vi "niRFUtil MASMT Mean (DBL).vi"(8 "error in (no error)":errorcluster, 11 "X":dbl[](array[numeric])) -> (0 "error out":errorcluster, 3 "mean":dbl)   [LabVIEW 2015, in "niRFUtil.lvlib"]
doc: "Computes the mean value of the input sequence <B>X</B>."
uses:
  niRFUtil.lvlib
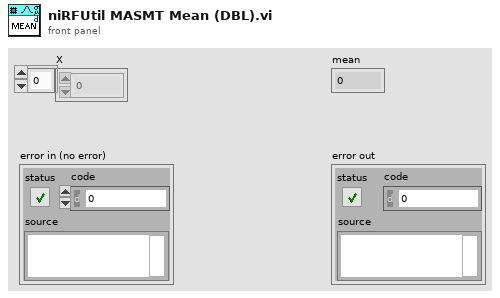
[diagram p1: front panel]
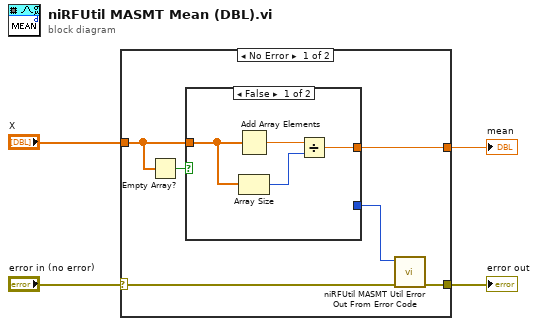
[diagram p0: block diagram]
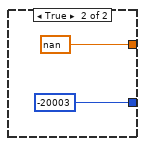
[diagram p2: hidden frame]
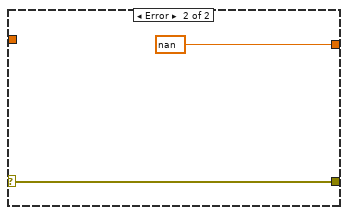
[diagram p3: hidden frame]
diagram:
  n1 = case shown="No Error" "error in (no error)" {
    selector: "error in (no error)" -> [w5 w17]
    tunnel: "X" -> [w9 _]
    tunnel: [w8 nan] -> w2
    tunnel: [w6 w17] -> w1
    frame No Error {
      n2 = Empty Array?(array=w9) -> (empty?=w10:bool)
      n3 = case shown="False" w10 {
        tunnel: w9 -> [w14 _]
        tunnel: [w11 nan] -> w8
        tunnel: [_ -20003] -> w7
        frame False {
          n4 = Add Array Elements(numeric array=w14) -> (sum=w13:dbl)
          n5 = Array Size(array=w14) -> (size(s)=w12:i32)
          n6 = Divide(x=w13, y=w12) -> (x/y=w11:dbl)
        }
        frame True {
        }
      }
      n7 = call "niRFUtil MASMT Util Error Out From Error Code.vi"("error in (no error)"=w5, "error code"=w7) -> ("error out"=w6:errorcluster)  [unwired: 9 in]
    }
    frame Error {
    }
  }
  "mean" <- w2
  "error out" <- w1
